vi "SelectData.vi"(8 "error in (no error)":errorcluster, 10 "Select Conditions Criteria":T1, 11 "object in":refnum<class "TableLogger_CSV_Actor.lvclass">) -> (0 "error out":errorcluster, 2 "Data Clusters":variant[](array[variant]), 3 "object out":refnum<class "TableLogger_CSV_Actor.lvclass">)   [LabVIEW 2014, in "TableLogger_CSV_Actor.lvlib" / "TableLogger_CSV_Actor.lvclass"]
uses:
  TableLogger_CSV_Actor.lvclass
  TableLogger_Actor/SelectConditionCriteria.ctl
  TableLogger_SQLite_Actor/SelectConditions.ctl
  TableLogger_CSV_Actor.lvclass/TableLogger_CSV_Actor.ctl
  TableLogger_Actor/TableLogger_Actor/TableLogger_Actor.lvclass
  TableLogger_SQLite_Actor/TableLogger_SQLite_Actor/TableLogger_SQLite_Actor.lvclass
  TableLogger_Actor/TableLogger_Actor.lvlib
panel:
  # "Connector Pane"
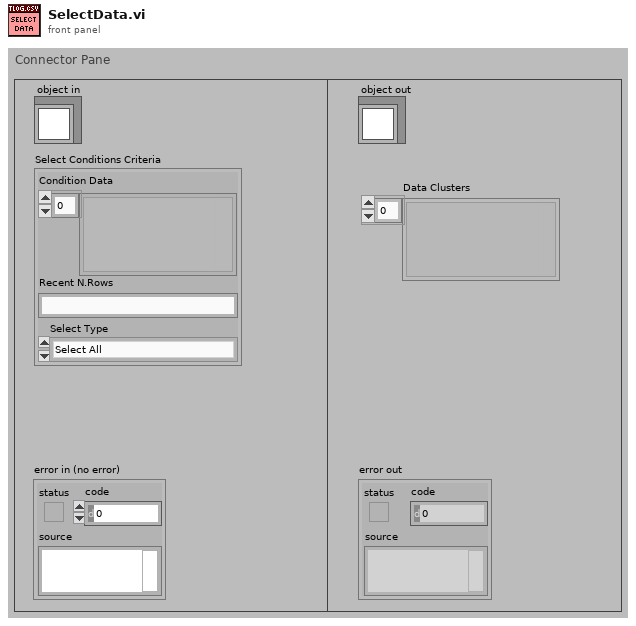
[diagram p1: front panel]
types:
  T1 = typedef "TableLogger_Actor.lvlib/SelectConditionCriteria.ctl" = cluster{"Condition Data":variant[], "Recent N.Rows":string, "Select Type":T2}
  T2 = typedef "TableLogger_Actor.lvlib/SelectConditions.ctl" = enum16{"Select All", "Select with AND Operator", "Select Most Recent Rows", "Select with OR Operator", "Select with BETWEEN Operator"}
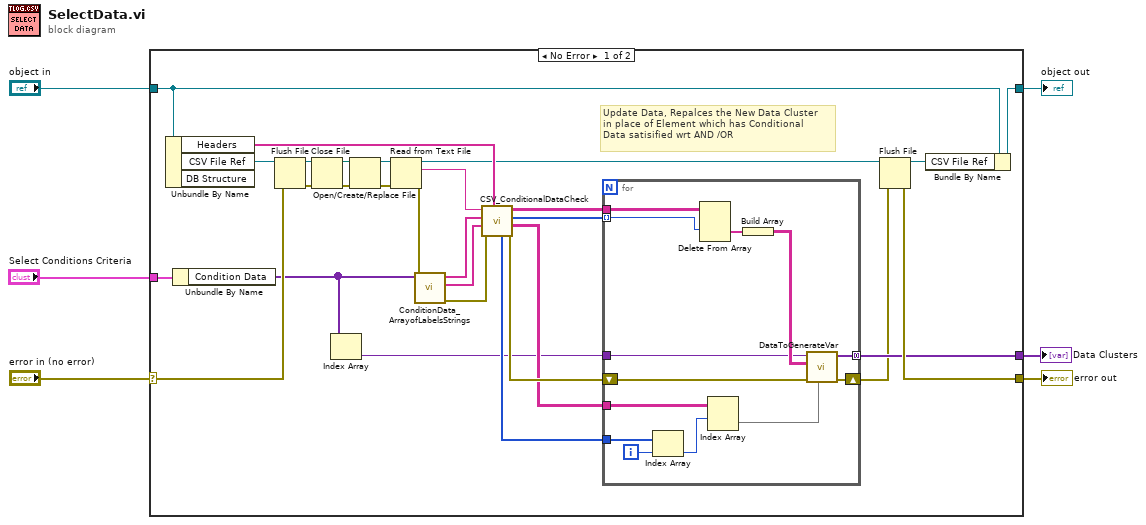
[diagram p0: block diagram]
diagram:
  n1 = case shown="No Error" "error in (no error)" {
    selector: "error in (no error)" -> [w34 w50]
    tunnel: [w32 w50] -> w6
    tunnel: [w29 w49] -> w4
    tunnel: "object in" -> [w30 w49]
    tunnel: [w20 _] -> w2
    tunnel: "Select Conditions Criteria" -> [w9 _]
    frame No Error {
      # "Update Data, Repalces the New Data Cluster\nin place of Element which has Conditional \nData satisified wrt AND /OR"
      n2 = Unbundle By Name(w30) -> ("Headers"=w22:string[], "CSV File Ref"=w33:refnum<file>)  [unwired: 1 out]
      n3 = Unbundle By Name(w9) -> ("Condition Data"=w8:variant[])
      n4 = Flush File(refnum=w33, error in=w34) -> (refnum out=w27:refnum<file>, error out=w25:errorcluster)
      n5 = Close File(refnum=w27, error in=w25) -> (path=w28:path, error out=w24:errorcluster)
      n6 = Index Array(array=w8) -> (element=w7:variant)  [unwired: 1 in]
      n7 = Open/Create/Replace File(file path (use dialog)=w28, error in=w24) -> (refnum out=w26:refnum<file>, error out=w23:errorcluster)  [unwired: 4 in, 1 out]
      n8 = Read from Text File(file (use dialog)=w26, error in=w23) -> (refnum out=w21:refnum<file>, text=w35:string, error out=w13:errorcluster)  [unwired: 2 in, 1 out]
      n9 = call "ConditionData_ArrayofLabelsStrings.vi"("error in (no error)"=w13, "Condition Data"=w8) -> ("error out"=w12:errorcluster, "Value"=w10:string[], "Label"=w11:string[])  [unwired: 7 in]
      n10 = call "CSV_ConditionalDataCheck.vi"("Headers"=w22, "error in"=w12, "A[Data]"=w10, "A[Labels]"=w11, "Data"=w35) -> ("error out"=w19:errorcluster, "Selected Headers"=w14:string[][], "Indexes for Conditional Data"=w15:i32[], "Data in 2D"=w17:string[][], "Seleted Indices"=w16:i32[])  [unwired: 2 in]
      n11 = for {
        tunnel: [w48] -> w20 mode=concatenating
        shift-right: [w46] -> w18
        shift-left: w19 -> [w47]
        tunnel: w16 -> [w40]
        tunnel: w15 -> [w44] mode=indexing
        tunnel: w14 -> [w41]
        tunnel: w17 -> [w45]
        tunnel: w7 -> [w36]
        i -> [w39]
        n12 = Index Array(array=w40, index=w39) -> (element=w38:i32)
        n13 = Delete From Array(array=w45, index (row)=w44) -> (deleted portion=w43:string[])  [unwired: 2 in, 1 out]
        n14 = Index Array(array=w41, index (row)=w38) -> (element=w37:string[])  [unwired: 1 in]
        n15 = Build Array(w43) -> (w42:string[][])
        n16 = call "DataToGenerateVar.vi"("Header"=w37, "error in (no error)"=w47, "Data in"=w42, "Variant"=w36) -> ("error out"=w46:errorcluster, "Data"=w48:variant[])  [unwired: 6 in]
      }
      n17 = Flush File(refnum=w21, error in=w18) -> (refnum out=w31:refnum<file>, error out=w32:errorcluster)
      n18 = Bundle By Name(cluster=w30, "CSV File Ref"=w31) -> (w29:refnum<class "TableLogger_CSV_Actor.lvclass">)
    }
    frame Error {
    }
  }
  "error out" <- w6
  "object out" <- w4
  "Data Clusters" <- w2
